vi "Signal_acquisition_v2.vi"() -> ()   [LabVIEW 2015]
uses:
  <vilib>/measure/matone.llb/Extract Single Tone Information 1 Chan.vi
  <vilib>/measure/madcrms.llb/Basic Averaged DC-RMS for 1 Chan.vi
  <vilib>/express/express arith-compare/Formula/XNode/ExpressFormulaBlockNode.xnode
  <vilib>/measure/NI_MAPro.lvlib
  <vilib>/Analysis/NI_AALPro.lvlib
panel:
  out "Cutoff Freqs (Hz)":i32[](array[numeric])
  out "Voltage Gain / Frequency":cluster{i32, dbl}[](graph)
  out "FRECUENCY END":i32
  out "FRECUENCY SWEEP":cluster{i32[], dbl[]}(graph)
  in  "FREQ START 5":i32
  in  "number of intervals  3":i32
  in  "number of intervals  2":i32
  in  "FREQ END":i32=70000
  in  "FREQ START":i32=10000
  in  "number \nof intervals":i32=60
  out "Time Shift":dbl
  out "magnitude":dbl
  out "Freq":dbl=0.3
  out "Phase Shift":dbl
  in  "SAVE DATA":bool
  out "RESULT \nin amplittude":dbl
  out "REFERENCE amplitude":dbl format="%.2p"
  in  "MEASURE AMPLITUD":bool
  in  "MEASURE PHASE":bool
  out "Phase":dbl(knob) scale=0.0..90.0
  out "detected \nphase (deg) 2":dbl format="%.2p"
  out "detected \nfrequency 2":dbl format="%.2p"
  out "DC value 2":dbl format="%0.2p"
  in  "input 2":u16=1
  in  "timeout ms":i32=2000
  out "REAL TIME MEASUREMENT":dbl[](graph)
  in  "Trigger Mode 2":string(combo)="CH1_NE"
  in  "Pause for buffer (ms) 2":u32=100
  in  "MEASURE REFERENCE":bool
  out "detected phase (deg)":dbl format="%.2p"
  out "detected frequency":dbl format="%.2p"
  out "MEASURED amplitud":dbl format="%.2p"
  in  "input 1":u16=1
  out "Acquisition\ntime complete":u32
  out "millisecond \nfinal timer":u32
  out "millisecond \nbegin timer":u32
  out "millisecond \ntimer value":u32
  out "Ieration number":i32
  in  "timeout ms\n (2000)":i32=2000
  in  "timeout ms\n (2000)":i32=2000
  in  "timeout ms\n (2000)":i32=2000
  out "error out":errorcluster
  out "WAVEFORM BASE LINE":dbl[](graph)
  in  "Trigger Mode":string(combo)="CH2_NE"
  in  "Pause for\n buffer (ms)":u32=100
  in  "Delay\n (# Samples)":i32 max=16348
  in  "Trigger Level \n(0 mV)":i32
  in  "IP address":string="161.111.10.6"
  in  "Decimation":u16(ring)=8 items=["65536"=65535, "8192"=8192, "1024"=1024, "64"=64, "16"=8, "1"=1]
  in  "error in":errorcluster
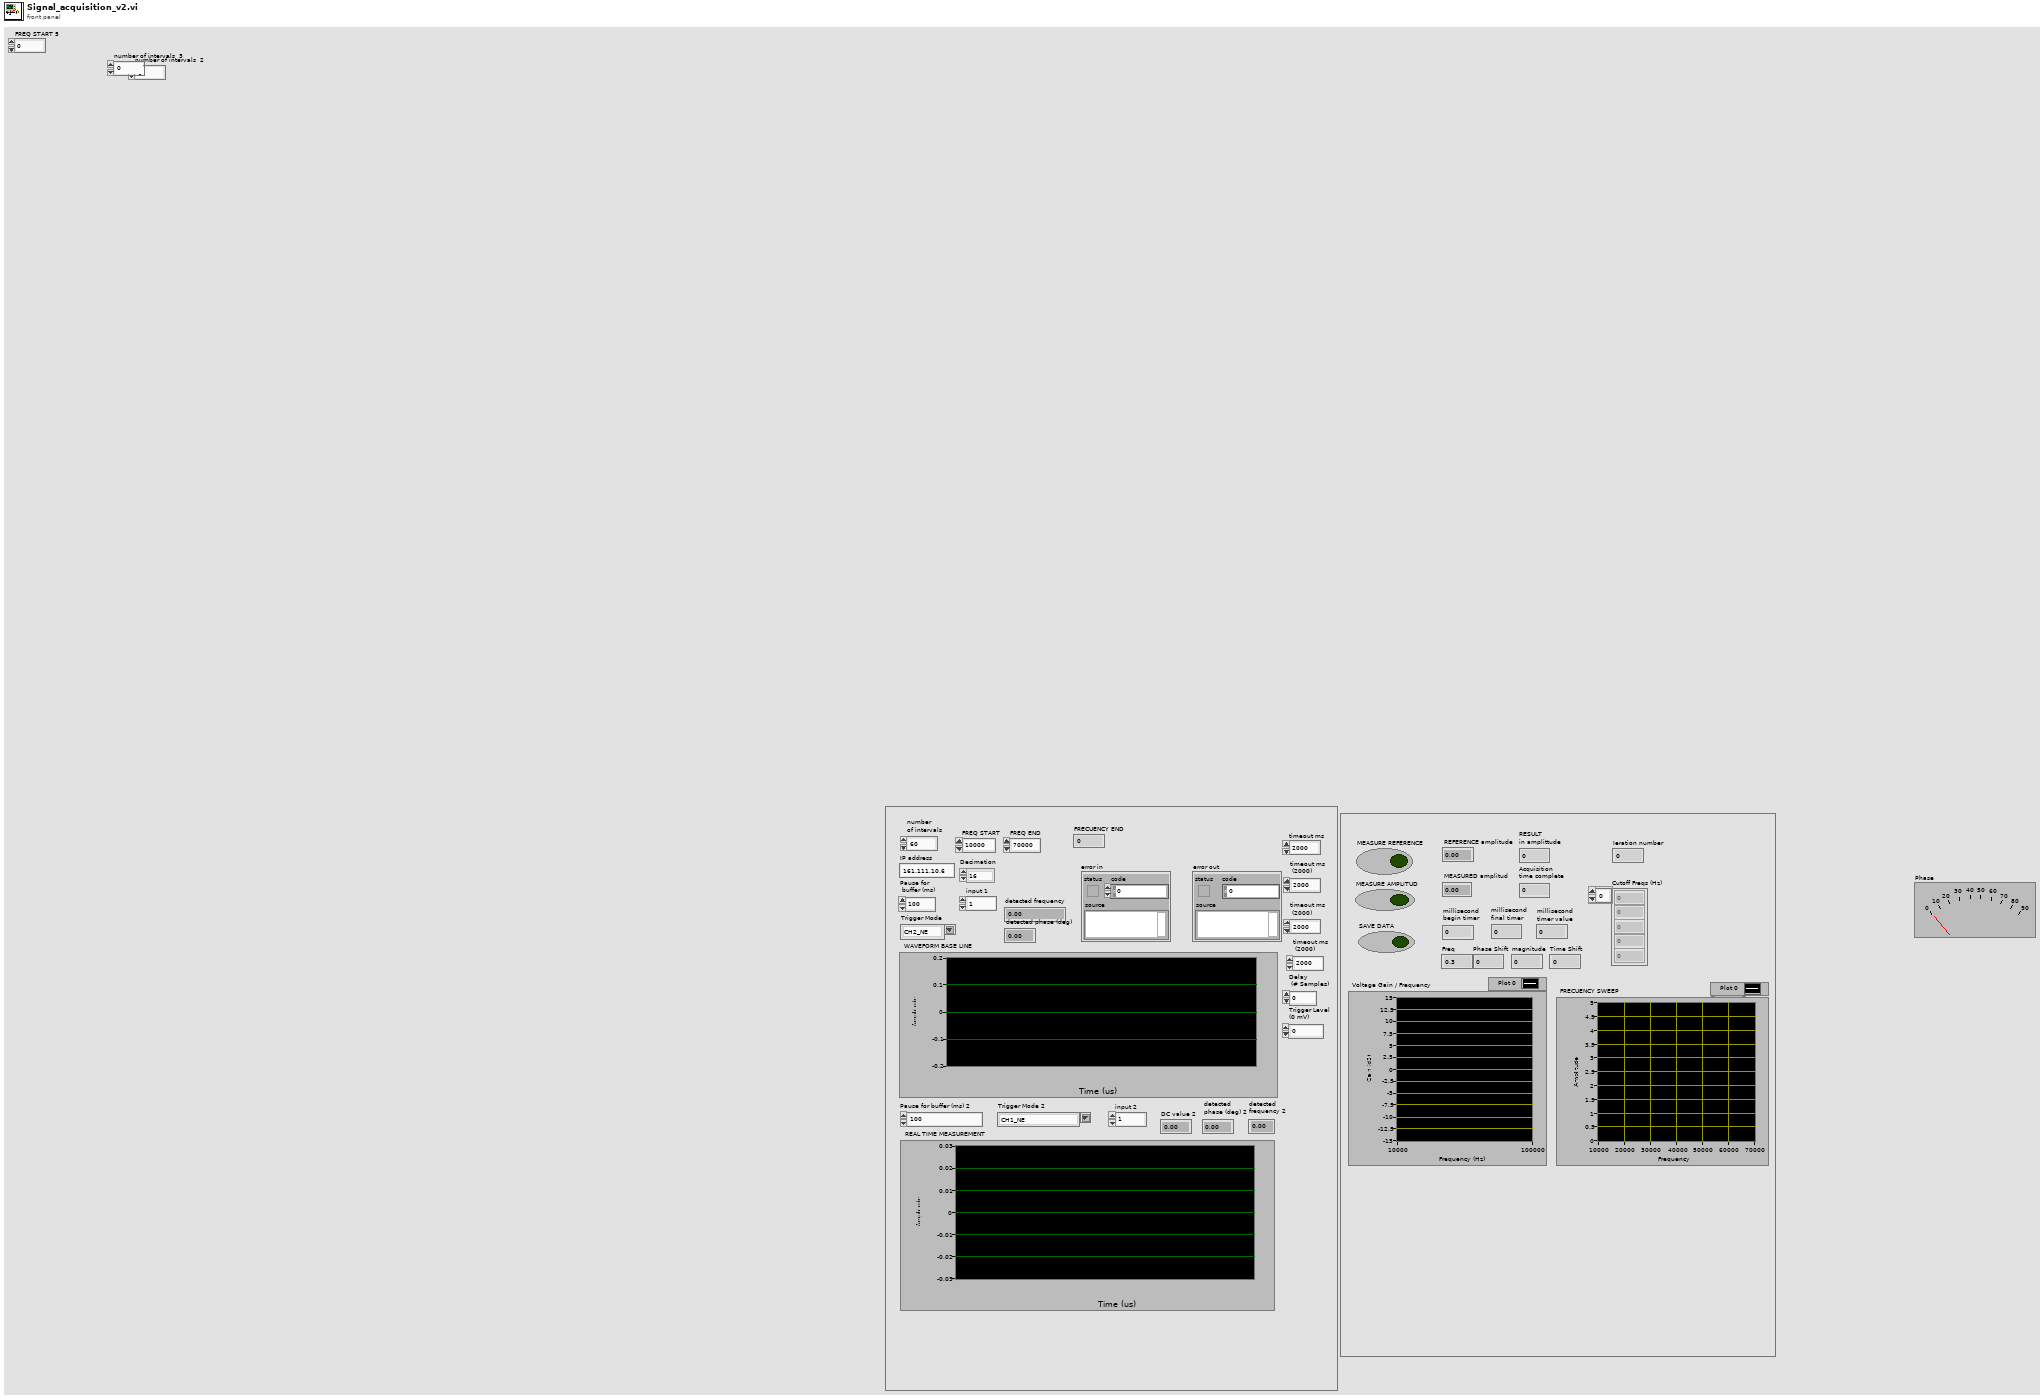
[diagram p1: front panel]
types:
  T1 = enum16{"Standard", "Buffered", "CRLF", "Immediate"}
  T2 = enum32{"none", "input signal", "detected signal", "residual signal"}
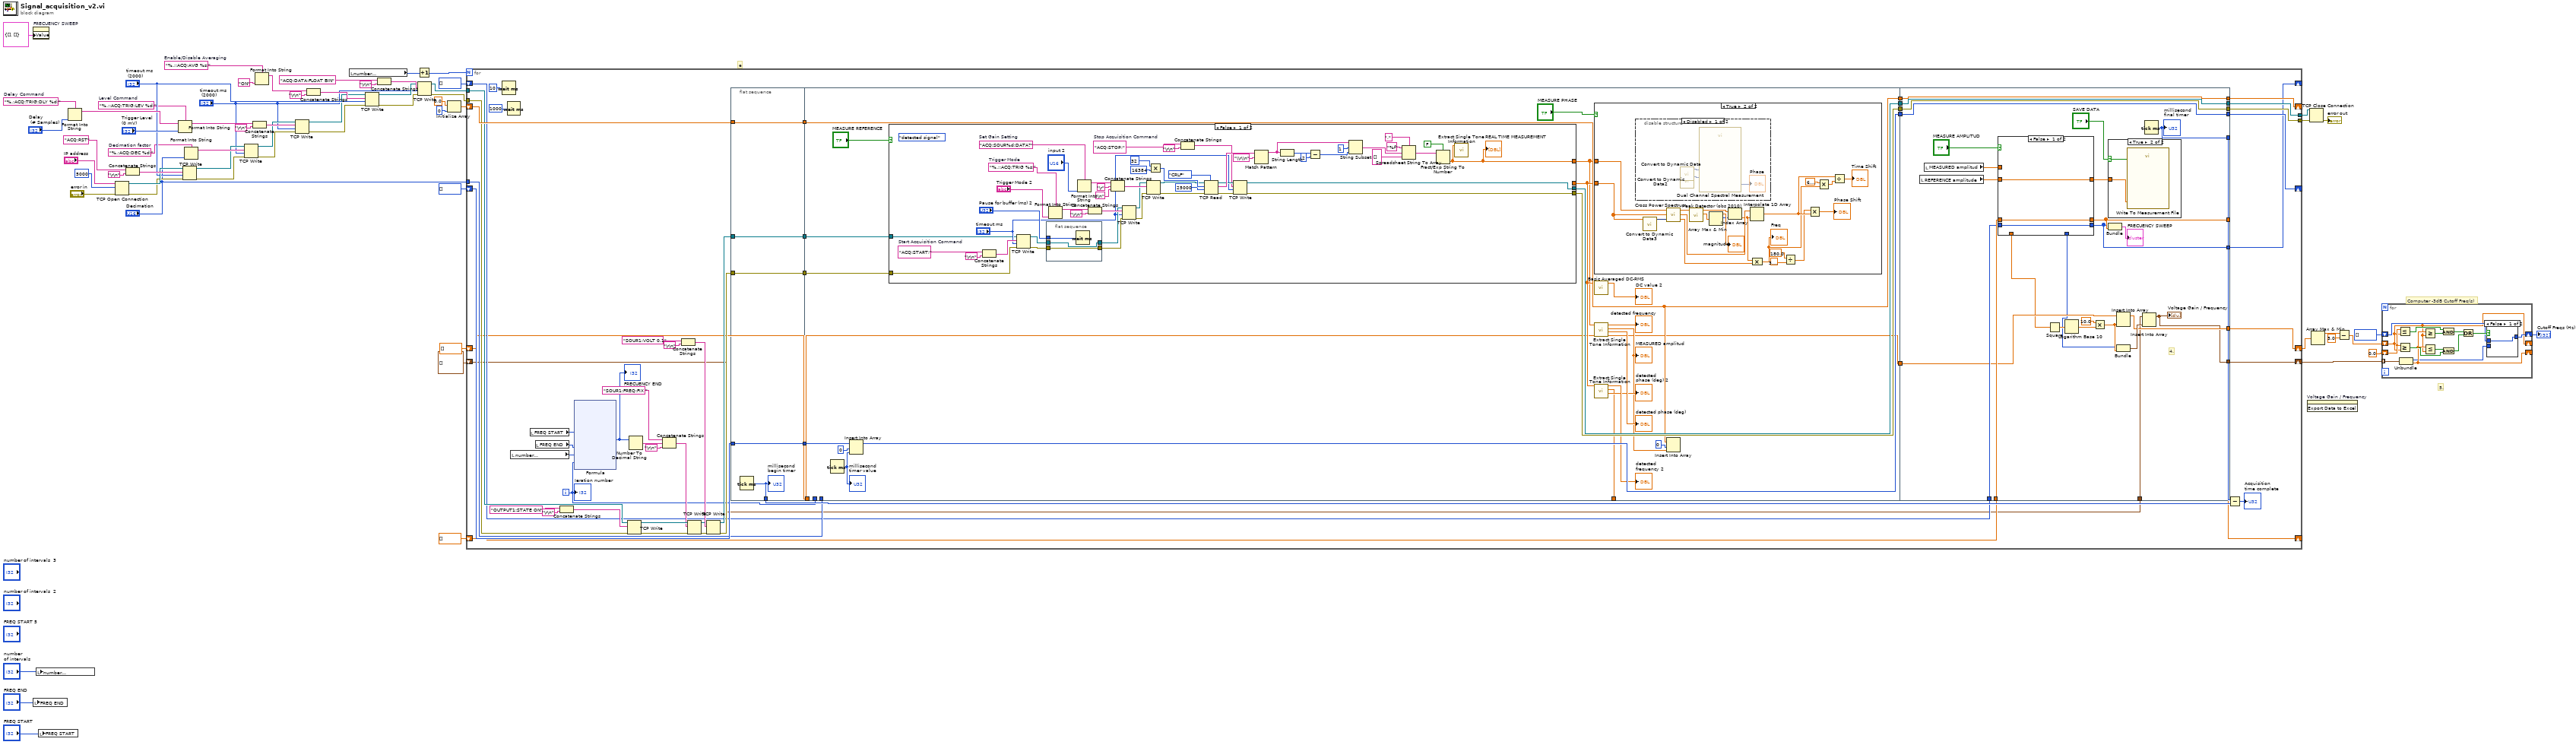
[diagram p0: block diagram]
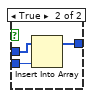
[diagram p2: hidden frame]
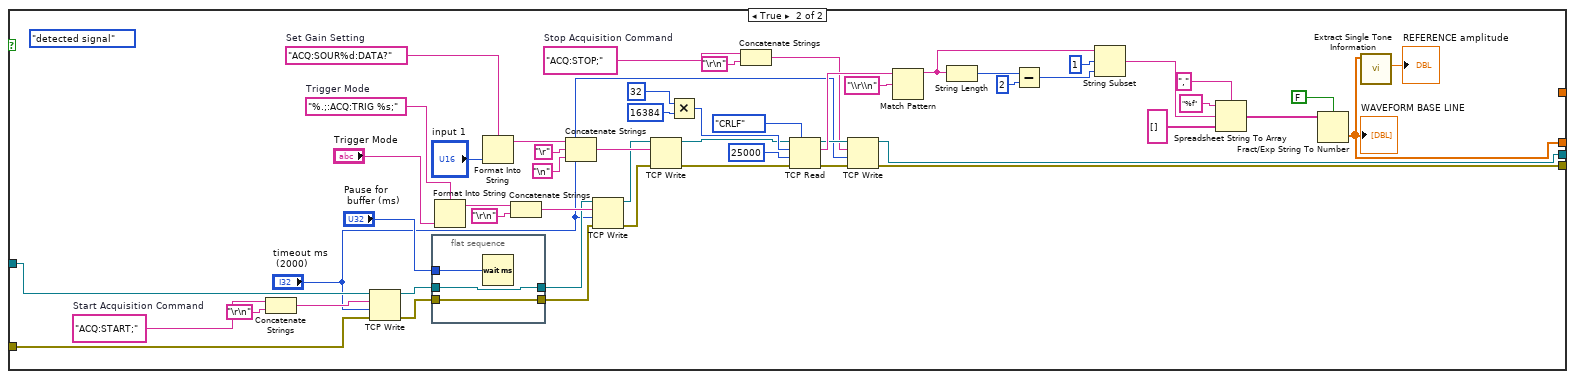
[diagram p5: hidden frame]
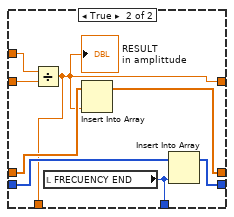
[diagram p7: hidden frame]
diagram:
  w30 = "%.;:ACQ:AVG %s;"  # Enable/Disable Averaging
  w38 = "%.;ACQ:DEC %d;"  # Decimation factor
  w39 = "%.;ACQ:TRIG:DLY %d;"  # Delay Command
  w40 = "%.;:ACQ:TRIG:LEV %d;"  # Level Command
  # "5."
  # "Computer -3dB Cutoff Freq(s)"
  # "e"
  n1 = property on="FRECUENCY SWEEP" class="XYGraph (strict)"("Value"=cluster{dbl[], dbl[]} {[], []} ("FRECUENCY SWEEP")) -> ()  [unwired: 2 in, 2 out]
  n2 = local write "FREQ END"("FREQ END") -> ()
  n3 = local write "number \nof intervals"("number \nof intervals") -> ()
  n4 = local write "FREQ START"("FREQ START") -> ()
  n5 = Format Into String(format string=w39, "Delay\n (# Samples)") -> (resulting string=w58:string)  [unwired: 2 in, 1 out]
  n6 = TCP Open Connection(address="IP address", remote port or service name=u16 5000, error in (no error)="error in") -> (connection ID=w52:refnum<k5>, error out=w51:errorcluster)  [unwired: 2 in]
  n7 = Concatenate Strings("ACQ:RST" ("SCPI Message"), "\r\n") -> (w54:string)
  n8 = Format Into String(format string=w40, initial string=w58, "Trigger Level \n(0 mV)") -> (resulting string=w55:string)  [unwired: 1 in, 1 out]
  n9 = TCP Write(connection ID=w52, data in=w54, error in (no error)=w51, 9:"timeout ms\n (2000)") -> (connection ID out=w36:refnum<k5>, error out=w35:errorcluster)  [unwired: 1 out]
  n10 = Format Into String(format string=w38, "Decimation") -> (resulting string=w37:string)  [unwired: 2 in, 1 out]
  n11 = TCP Write(connection ID=w36, data in=w37, error in (no error)=w35, 9:"timeout ms\n (2000)") -> (connection ID out=w34:refnum<k5>, error out=w33:errorcluster)  [unwired: 1 out]
  n12 = Concatenate Strings(w55, "\r\n") -> (w49:string)
  n13 = Format Into String(format string=w30, "ON") -> (resulting string=w61:string)  [unwired: 2 in, 1 out]
  n14 = TCP Write(connection ID=w34, data in=w49, error in (no error)=w33, 9:"timeout ms\n (2000)") -> (connection ID out=w32:refnum<k5>, error out=w31:errorcluster)  [unwired: 1 out]
  n15 = Concatenate Strings(w61, "\r\n") -> (w50:string)
  n16 = local read "number \nof intervals"() -> (w16:i32)
  n17 = TCP Write(connection ID=w32, data in=w50, error in (no error)=w31, 9:"timeout ms\n (2000)") -> (connection ID out=w28:refnum<k5>, error out=w27:errorcluster)  [unwired: 1 out]
  n18 = Concatenate Strings("ACQ:DATA:FLOAT BIN" ("SCPI Message"), "\r\n") -> (w46:string)
  n19 = Increment(x=w16) -> (x+1=w15:i32)
  n20 = TCP Write(connection ID=w28, data in=w46, error in (no error)=w27, 9:"timeout ms\n (2000)") -> (connection ID out=w25:refnum<k5>, error out=w24:errorcluster)  [unwired: 1 out]
  n21 = Initialize Array(0.0 ("element"), 0 ("dimension size")) -> (w19:dbl[])
  n22 = for {
    N: w15 -> [_]
    tunnel: w25 -> [w86]
    tunnel: [w114] -> w45
    tunnel: [w113] -> w44
    tunnel: w24 -> [w83]
    shift-right: [w116] -> _
    shift-left: u32[] [] -> [w115]
    tunnel: "Decimation" -> [w103]
    shift-right: [w100] -> _
    shift-left: w19 -> [w98]
    shift-right: [w79] -> _
    shift-left: dbl[] [] -> [w80]
    shift-right: [w75] -> _
    shift-left: i32[] [] -> [w74]
    shift-right: [w69] -> w3
    shift-left: dbl[] [] -> [w67]
    shift-right: [w66] -> w2
    shift-left: cluster{"FRECUENCY END":i32, dbl}[] [] -> [w65]
    i -> [w73]
    n23 = Wait (ms)(milliseconds to wait=u32 10) -> ()  [unwired: 1 out]
    n24 = Wait (ms)(milliseconds to wait=u32 1000) -> ()  [unwired: 1 out]
    n25 = local read "number \nof intervals"() -> (w76:i32)
    n26 = local read "FREQ START"() -> (w77:i32)
    n27 = local read "FREQ END"() -> (w78:i32)
    n28 = Concatenate Strings("OUTPUT1:STATE ON" ("SCPI Message"), "\r\n") -> (w96:string)
    n29 = xnode "Formula"("Fin"=w77, "Fend"=w78, "Ninter"=w76, "i"=w73) -> ("Result"=w70:i32)  [unwired: 1 in, 1 out]
    "FRECUENCY END" <- w70
    n30 = TCP Write(connection ID=w86, data in=w96, error in (no error)=w83) -> (connection ID out=w93:refnum<k5>, error out=w92:errorcluster)  [unwired: 1 in, 1 out]
    n31 = Number To Decimal String(number=w70) -> (decimal integer string=w81:string)  [unwired: 1 in]
    n32 = Concatenate Strings("SOUR1:FREQ:FIX " ("SCPI Message"), w81, "\r\n") -> (w88:string)
    n33 = Concatenate Strings("SOUR1:VOLT 0.1" ("SCPI Message"), "\r\n") -> (w87:string)
    n34 = TCP Write(connection ID=w93, data in=w88, error in (no error)=w92) -> (connection ID out=w72:refnum<k5>, error out=w71:errorcluster)  [unwired: 1 in, 1 out]
    n35 = TCP Write(connection ID=w72, data in=w87, error in (no error)=w71) -> (connection ID out=w85:refnum<k5>, error out=w84:errorcluster)  [unwired: 1 in, 1 out]
    n36 = flat-sequence {
      tunnel: w115 -> [w133]
      tunnel: w84 -> [w134]
      tunnel: w85 -> [w135]
      tunnel: [w135] -> w109
      tunnel: [w134] -> w108
      tunnel: [w133] -> w107
      tunnel: [w132] -> w105
      tunnel: [w131] -> w99
      tunnel: w98 -> [w131]
      tunnel: [w153] -> w112
      tunnel: [w151] -> w111
      tunnel: [w150] -> w110
      tunnel: w109 -> [w157]
      tunnel: w108 -> [w156]
      tunnel: w107 -> [w152]
      tunnel: w103 -> [_]
      tunnel: [w146] -> w101
      tunnel: w73 -> [_]
      tunnel: w99 -> [w146]
      tunnel: [w137] -> _
      tunnel: w67 -> [w136]
      tunnel: [w136] -> w68
      tunnel: [w315] -> w113
      tunnel: [w316] -> w114
      tunnel: [w317] -> w116
      tunnel: w112 -> [w317]
      tunnel: w111 -> [w316]
      tunnel: w110 -> [w315]
      tunnel: [w314] -> w106
      tunnel: w101 -> [w313]
      tunnel: [w313] -> w100
      tunnel: w80 -> [w307]
      tunnel: [w305] -> w79
      tunnel: [w304] -> w75
      tunnel: w74 -> [w306]
      tunnel: [w297] -> w69
      tunnel: w68 -> [w296]
      tunnel: [w293] -> w66
      tunnel: w65 -> [w292]
      frame #0 {
        n37 = Tick Count (ms)() -> (millisecond timer value=w132:u32)
        "millisecond \nbegin timer" <- w132
      }
      frame #1 {
        n38 = Tick Count (ms)() -> (millisecond timer value=w154:u32)
        "millisecond \ntimer value" <- w154
        n39 = Insert Into Array(array=w152, index=0, new element=w154) -> (w153:u32[])
        n40 = case shown="False" "MEASURE REFERENCE" {
          tunnel: w157 -> [w182 w285]
          tunnel: w156 -> [w185 w249]
          tunnel: [w183 w246] -> w151
          tunnel: [w184 w241] -> w150
          tunnel: [w181 _] -> w139
          tunnel: [_ w237] -> w141
          frame False {
            w192 = "ACQ:STOP;"  # Stop Acquisition Command
            (unwired) T2."detected signal" ("export mode")
            w202 = "ACQ:SOUR%d:DATA?"  # Set Gain Setting
            w229 = "%.;:ACQ:TRIG %s;"  # Trigger Mode
            w231 = "ACQ:START;"  # Start Acquisition Command
            n41 = Concatenate Strings(w231, "\r\n") -> (w232:string)
            n42 = TCP Write(connection ID=w182, data in=w232, error in (no error)=w185, 9:"timeout ms") -> (connection ID out=w206:refnum<k5>, error out=w205:errorcluster)  [unwired: 1 out]
            n43 = flat-sequence {
              tunnel: "Pause for buffer (ms) 2" -> [w235]
              tunnel: [w234] -> w204
              tunnel: [w233] -> w203
              tunnel: w206 -> [w234]
              tunnel: w205 -> [w233]
              frame #0 {
                n44 = Wait (ms)(milliseconds to wait=w235) -> ()  [unwired: 1 out]
              }
            }
            n45 = Format Into String(format string=w229, "Trigger Mode 2") -> (resulting string=w226:string)  [unwired: 2 in, 1 out]
            n46 = Format Into String(format string=w202, "input 2") -> (resulting string=w200:string)  [unwired: 2 in, 1 out]
            n47 = Concatenate Strings(w226, "\r\n") -> (w227:string)
            n48 = Concatenate Strings(w200, "\r", "\n") -> (w199:string)
            n49 = TCP Write(connection ID=w204, data in=w227, error in (no error)=w203, 9:"timeout ms") -> (connection ID out=w197:refnum<k5>, error out=w196:errorcluster)  [unwired: 1 out]
            n50 = TCP Write(connection ID=w197, data in=w199, error in (no error)=w196) -> (connection ID out=w198:refnum<k5>, error out=w195:errorcluster)  [unwired: 1 in, 1 out]
            n51 = Multiply(x=32, y=16384 ("bytes to read")) -> (x*y=w207:i32)
            n52 = Concatenate Strings(w192, "\r\n") -> (w190:string)
            n53 = TCP Read(connection ID=w198, bytes to read=w207, error in (no error)=w195, 7:T1."CRLF" ("mode (standard)"), 9:25000 ("timeout ms (25000)")) -> (connection ID out=w193:refnum<k5>, data out=w208:string, error out=w189:errorcluster)
            n54 = TCP Write(connection ID=w193, data in=w190, error in (no error)=w189, 9:"timeout ms") -> (connection ID out=w183:refnum<k5>, error out=w184:errorcluster)  [unwired: 1 out]
            n55 = Match Pattern(string=w208, regular expression="\\r\\n") -> (before substring=w214:string)  [unwired: 1 in, 3 out]
            n56 = String Length(string=w214) -> (length=w217:i32)
            n57 = Subtract(x=w217, y=2) -> (x-y=w218:i32)
            n58 = String Subset(string=w214, offset (0)=1, length (rest)=w218) -> (substring=w215:string)
            n59 = Spreadsheet String To Array(delimiter (Tab)=",", format string="%f", spreadsheet string=w215, array type (2D Dbl)=string[] [] ("Array")) -> (array=w221:string[])
            n60 = Fract/Exp String To Number(use system decimal point (T)=FALSE, string=w221) -> (number=w181:dbl[])  [unwired: 3 out]
            "REAL TIME MEASUREMENT" <- w181
            n61 = call-poly <vilib>:"Extract Single Tone Information.vi"("time signal in"=w181) -> ()  [unwired: 5 in, 6 out]
          }
          frame True {
            w245 = "ACQ:STOP;"  # Stop Acquisition Command
            (unwired) T2."detected signal" ("export mode")
            w257 = "ACQ:SOUR%d:DATA?"  # Set Gain Setting
            w284 = "%.;:ACQ:TRIG %s;"  # Trigger Mode
            w287 = "ACQ:START;"  # Start Acquisition Command
            n62 = Concatenate Strings(w287, "\r\n") -> (w288:string)
            n63 = TCP Write(connection ID=w285, data in=w288, error in (no error)=w249, 9:"timeout ms\n (2000)") -> (connection ID out=w261:refnum<k5>, error out=w260:errorcluster)  [unwired: 1 out]
            n64 = flat-sequence {
              tunnel: "Pause for\n buffer (ms)" -> [w291]
              tunnel: [w290] -> w259
              tunnel: [w289] -> w258
              tunnel: w261 -> [w290]
              tunnel: w260 -> [w289]
              frame #0 {
                n65 = Wait (ms)(milliseconds to wait=w291) -> ()  [unwired: 1 out]
              }
            }
            n66 = Format Into String(format string=w284, "Trigger Mode") -> (resulting string=w281:string)  [unwired: 2 in, 1 out]
            n67 = Format Into String(format string=w257, "input 1") -> (resulting string=w255:string)  [unwired: 2 in, 1 out]
            n68 = Concatenate Strings(w281, "\r\n") -> (w282:string)
            n69 = Concatenate Strings(w255, "\r", "\n") -> (w254:string)
            n70 = TCP Write(connection ID=w259, data in=w282, error in (no error)=w258, 9:"timeout ms\n (2000)") -> (connection ID out=w252:refnum<k5>, error out=w251:errorcluster)  [unwired: 1 out]
            n71 = TCP Write(connection ID=w252, data in=w254, error in (no error)=w251) -> (connection ID out=w253:refnum<k5>, error out=w250:errorcluster)  [unwired: 1 in, 1 out]
            n72 = Multiply(x=32, y=16384 ("bytes to read")) -> (x*y=w262:i32)
            n73 = Concatenate Strings(w245, "\r\n") -> (w243:string)
            n74 = TCP Read(connection ID=w253, bytes to read=w262, error in (no error)=w250, 7:T1."CRLF" ("mode (standard)"), 9:25000 ("timeout ms (25000)")) -> (connection ID out=w247:refnum<k5>, data out=w263:string, error out=w242:errorcluster)
            n75 = TCP Write(connection ID=w247, data in=w243, error in (no error)=w242, 9:"timeout ms\n (2000)") -> (connection ID out=w246:refnum<k5>, error out=w241:errorcluster)  [unwired: 1 out]
            n76 = Match Pattern(string=w263, regular expression="\\r\\n") -> (before substring=w269:string)  [unwired: 1 in, 3 out]
            n77 = String Length(string=w269) -> (length=w272:i32)
            n78 = Subtract(x=w272, y=2) -> (x-y=w273:i32)
            n79 = String Subset(string=w269, offset (0)=1, length (rest)=w273) -> (substring=w270:string)
            n80 = Spreadsheet String To Array(delimiter (Tab)=",", format string="%f", spreadsheet string=w270, array type (2D Dbl)=string[] [] ("Array")) -> (array=w276:string[])
            n81 = Fract/Exp String To Number(use system decimal point (T)=FALSE, string=w276) -> (number=w237:dbl[])  [unwired: 3 out]
            "WAVEFORM BASE LINE" <- w237
            n82 = call-poly <vilib>:"Extract Single Tone Information.vi"("time signal in"=w237) -> ("detected amplitude"=→"REFERENCE amplitude":dbl)  [unwired: 5 in, 5 out]
          }
        }
        n83 = case shown="True" "MEASURE PHASE" {
          tunnel: w139 -> [_ w160]
          tunnel: w141 -> [_ w158]
          frame False {
          }
          frame True {
            n84 = disable-structure shown="Disabled" {
              frame Disabled {
                n85 = call "Convert to Dynamic Data"() -> ("Dynamic Data Type"=w180:dynamicdata)  [unwired: 4 in]
                n86 = call "Convert to Dynamic Data2"() -> ("Dynamic Data Type"=w178:dynamicdata)  [unwired: 4 in]
                n87 = call "Dual Channel Spectral Measurement"("Input Signal B"=w178, "Input Signal A"=w180) -> ("Phase"=→"Phase":dynamicdata)  [unwired: 8 in, 1 out]
              }
              frame Enabled {
              }
            }
            n88 = call "Convert to Dynamic Data3"("Array"=w158) -> ("Dynamic Data Type"=w159:dynamicdata)  [unwired: 3 in]
            n89 = call <vilib>:"Cross Power Spectrum.vi"("dt"=w159, "Signal Y (V)"=w158, "Signal X (V)"=w160) -> ("df"=w174:dbl, "Cross Power XY Spectrum Phase (radians)"=w175:dbl[], "Cross Power XY Spectrum Mag (V^2rms)"=w173:dbl[])
            n90 = call <vilib>:"Peak Detector (obs 2010).vi"("X"=w173) -> ("Amplitudes"=w163:dbl[], "Locations"=w172:dbl[])  [unwired: 6 in, 3 out]
            n91 = Array Max & Min(array=w163) -> (max value=→"magnitude":dbl, max index (indices)=w162:i32)  [unwired: 2 out]
            n92 = Index Array(array=w172, index=w162) -> (element=w161:dbl)
            n93 = Interpolate 1D Array(1:w161, 2:w175) -> (0:w170:dbl)
            n94 = Compound Arithmetic op=MULTIPLY(w161, w174) -> (w168:dbl)
            "Freq" <- w168
            n95 = Divide(x=180.0, y=3.141592653589793) -> (x/y=w164:dbl)
            n96 = Multiply(x=w164, y=w170) -> (x*y=→"Phase Shift":dbl)
            n97 = Multiply(x=6.283185307179586, y=w168) -> (x*y=w167:dbl)
            n98 = Divide(x=w170, y=w167) -> (x/y=→"Time Shift":dbl)
          }
        }
        n99 = call-poly <vilib>:"Basic Averaged DC-RMS.vi"("signal in"=w141) -> ("DC value"=→"DC value 2":dbl)  [unwired: 7 in, 3 out]
        n100 = call-poly <vilib>:"Extract Single Tone Information.vi"("time signal in"=w139) -> ("detected phase (deg)"=→"detected phase (deg)":dbl, "detected amplitude"=w138:dbl, "detected frequency"=→"detected frequency":dbl)  [unwired: 5 in, 3 out]
        "MEASURED amplitud" <- w138
        n101 = call-poly <vilib>:"Extract Single Tone Information.vi"("time signal in"=w141) -> ("detected phase (deg)"=→"detected \nphase (deg) 2":dbl, "detected amplitude"=w137:dbl, "detected frequency"=→"detected \nfrequency 2":dbl)  [unwired: 5 in, 3 out]
        n102 = Insert Into Array(array=w146, index=0, new element=w138) -> ()  [unwired: 1 out]
      }
      frame #2 {
        # "4."
        n103 = local read "REFERENCE amplitude"() -> (w312:dbl)
        n104 = local read "MEASURED amplitud"() -> (w311:dbl)
        n105 = case shown="False" "MEASURE AMPLITUD" {
          tunnel: w312 -> [w322 w326]
          tunnel: w311 -> [_ w325]
          tunnel: [w322 w324] -> w309
          tunnel: w307 -> [w321 w330]
          tunnel: [w321 w329] -> w305
          tunnel: [w320 w328] -> w304
          tunnel: w306 -> [w320 w327]
          tunnel: [_ w324] -> w295
          tunnel: [_ w323] -> w294
          frame False {
          }
          frame True {
            n106 = Divide(x=w325, y=w326) -> (x/y=w324:dbl)
            "RESULT \nin amplittude" <- w324
            n107 = local read "FRECUENCY END"() -> (w323:i32)
            n108 = Insert Into Array(array=w330, new element=w324) -> (w329:dbl[])  [unwired: 1 in]
            n109 = Insert Into Array(array=w327, new element=w323) -> (w328:i32[])  [unwired: 1 in]
          }
        }
        n110 = Square(x=w295) -> (x^2=w299:dbl)
        n111 = Logarithm Base 10(1:w299) -> (0:w300:dbl)
        n112 = Multiply(x=10.0, y=w300) -> (x*y=w298:dbl)
        n113 = case shown="True" "SAVE DATA" {
          selector: "SAVE DATA" -> [_ w318]
          tunnel: w309 -> [_ w319]
          frame False {
          }
          frame True {
            n114 = call "Write To Measurement File"("Signals"=w319, "Enable"=w318) -> ()  [unwired: 15 in, 3 out]
          }
        }
        n115 = Bundle(w304, w305) -> (→"FRECUENCY SWEEP":cluster{i32[], dbl[]})  [unwired: 1 in]
        n116 = Insert Into Array(array=w296, new element=w298) -> (w297:dbl[])  [unwired: 1 in]
        n117 = Bundle("FRECUENCY END"=w294, w298) -> (w302:cluster{"FRECUENCY END":i32, dbl})  [unwired: 1 in]
        n118 = Insert Into Array(array=w292, new element=w302) -> (w293:cluster{"FRECUENCY END":i32, dbl}[])  [unwired: 1 in]
        "Voltage Gain / Frequency" <- w293
        n119 = Tick Count (ms)() -> (millisecond timer value=w314:u32)
        "millisecond \nfinal timer" <- w314
      }
    }
    n120 = Subtract(x=w106, y=w105) -> (x-y=→"Acquisition\ntime complete":u32)
    "Ieration number" <- w73
  }
  n121 = invoke on="Voltage Gain / Frequency" class="XYGraph (strict)" method="Export Data to Excel"() -> ()  [unwired: 3 in, 3 out]
  n122 = TCP Close Connection(connection ID=w45, error in (no error)=w44) -> (error out=→"error out":errorcluster)  [unwired: 1 in, 1 out]
  n123 = Array Max & Min(array=w3) -> (max value=w4:dbl)  [unwired: 3 out]
  n124 = Subtract(x=w4, y=3.0) -> (x-y=w5:dbl)
  n125 = for {
    tunnel: w2 -> [w344] mode=indexing
    shift-right: [w338] -> _
    shift-left: 0.0 -> [w339]
    shift-right: [w332] -> w7
    shift-left: i32[] [] -> [w333]
    shift-right: [w331] -> _
    shift-left: w5 -> [w331]
    n126 = Less Or Equal?(x=w339, y=w331) -> (x <= y?=w342:bool)
    n127 = Greater Or Equal?(x=w339, y=w331) -> (x >= y?=w340:bool)
    n128 = Unbundle(w344) -> ("FRECUENCY END"=w334:i32, w338:dbl)
    n129 = Greater Or Equal?(x=w338, y=w331) -> (x >= y?=w343:bool)
    n130 = Less Or Equal?(x=w338, y=w331) -> (x <= y?=w341:bool)
    n131 = And(x=w342, y=w343) -> (x .and. y?=w336:bool)
    n132 = And(x=w341, y=w340) -> (x .and. y?=w337:bool)
    n133 = Or(x=w336, y=w337) -> (x .or. y?=w335:bool)
    n134 = case shown="False" w335 {
      tunnel: w334 -> [_ w348]
      tunnel: w333 -> [w345 w347]
      tunnel: [w345 w346] -> w332
      frame False {
      }
      frame True {
        n135 = Insert Into Array(array=w347, new element=w348) -> (w346:i32[])  [unwired: 1 in]
      }
    }
  }
  "Cutoff Freqs (Hz)" <- w7
